vi "rsscope_core_global.vi"() -> ()   [LabVIEW 2014] (continued)
"Data Type"=0, "Command"="BUS{SerialBus}:DPHY:DPTW:SOUR", "Access"=2, "Range Table"="rsscope_rngWaveformParameter", "Read Callback"="", "Write Callback"="", "Supported Models"="", "Instrument Options"="K42", "Flags"=0, "Help"="Selects the source of the high speed data lane.\n\nAvailable Repeated Capabilities:\nSerialBus: SB1, SB2, SB3, SB4\r\n\nRemote-control command(s):\nBUS<m>:DPHY:DPTWo:SOURce"}, {"Level"=3, "Class Only"=FALSE, "Identifier"="RSSCOPE_ATTR_PROTOCOL_DPHY_DP_THREE_SOURCE", "Descriptive Name"="Protocol DPHY DP Three Source", "Data Type"=0, "Command"="BUS{SerialBus}:DPHY:DPTH:SOUR", "Access"=2, "Range Table"="rsscope_rngWaveformParameter", "Read Callback"="", "Write Callback"="", "Supported Models"="", "Instrument Options"="K42", "Flags"=0, "Help"="Selects the source of the high speed data lane.\n\nAvailable Repeated Capabilities:\nSerialBus: SB1, SB2, SB3, SB4\r\n\nRemote-control command(s):\nBUS<m>:DPHY:DPTHree:SOURce"}, {"Level"=3, "Class Only"=FALSE, "Identifier"="RSSCOPE_ATTR_PROTOCOL_DPHY_CP_PROBE", "Descriptive Name"="Protocol DPHY CP Probe", "Data Type"=0, "Command"="BUS{SerialBus}:DPHY:CP:PROB", "Access"=2, "Range Table"="rsscope_rngProbeDisplayDiff", "Read Callback"="", "Write Callback"="", "Supported Models"="", "Instrument Options"="", "Flags"=0, "Help"="Selects the type of probe used for the clock lane.\n\nAvailable Repeated Capabilities:\nSerialBus: SB1, SB2, SB3, SB4\r\n\nRemote-control command(s):\nBUS<m>:DPHY:CP:PROBe"}, {"Level"=3, "Class Only"=FALSE, "Identifier"="RSSCOPE_ATTR_PROTOCOL_DPHY_DN_ZERO_PROBE", "Descriptive Name"="Protocol DPHY DN Zero Probe", "Data Type"=0, "Command"="BUS{SerialBus}:DPHY:DNZ:PROB", "Access"=2, "Range Table"="rsscope_rngProbeDisplayDiff", "Read Callback"="", "Write Callback"="", "Supported Models"="", "Instrument Options"="K42", "Flags"=0, "Help"="Selects the type of probe used for the corresponding data lane.\n\nAvailable Repeated Capabilities:\nSerialBus: SB1, SB2, SB3, SB4\r\n\nRemote-control command(s):\nBUS<m>:DPHY:DNZero:PROBe"}, {"Level"=3, "Class Only"=FALSE, "Identifier"="RSSCOPE_ATTR_PROTOCOL_DPHY_DP_ZERO_PROBE", "Descriptive Name"="Protocol DPHY DP Zero Probe", "Data Type"=0, "Command"="BUS{SerialBus}:DPHY:DPZ:PROB", "Access"=2, "Range Table"="rsscope_rngProbeDisplayDiff", "Read Callback"="", "Write Callback"="", "Supported Models"="", "Instrument Options"="K42", "Flags"=0, "Help"="Selects the type of probe used for the corresponding data lane.\n\nAvailable Repeated Capabilities:\nSerialBus: SB1, SB2, SB3, SB4\r\n\nRemote-control command(s):\nBUS<m>:DPHY:DPZero:PROBe"}, {"Level"=3, "Class Only"=FALSE, "Identifier"="RSSCOPE_ATTR_PROTOCOL_DPHY_DP_ONE_PROBE", "Descriptive Name"="Protocol DPHY DP One Probe", "Data Type"=0, "Command"="BUS{SerialBus}:DPHY:DPON:PROB", "Access"=2, "Range Table"="rsscope_rngProbeDisplayDiff", "Read Callback"="", "Write Callback"="", "Supported Models"="", "Instrument Options"="K42", "Flags"=0, "Help"="Selects the type of probe used for the corresponding data lane.\n\nAvailable Repeated Capabilities:\nSerialBus: SB1, SB2, SB3, SB4\r\n\nRemote-control command(s):\nBUS<m>:DPHY:DPONe:PROBe"}, {"Level"=3, "Class Only"=FALSE, "Identifier"="RSSCOPE_ATTR_PROTOCOL_DPHY_DP_TWO_PROBE", "Descriptive Name"="Protocol DPHY DP Two Probe", "Data Type"=0, "Command"="BUS{SerialBus}:DPHY:DPTW:PROB", "Access"=2, "Range Table"="rsscope_rngProbeDisplayDiff", "Read Callback"="", "Write Callback"="", "Supported Models"="", "Instrument Options"="K42", "Flags"=0, "Help"="Selects the type of probe used for the corresponding data lane.\n\nAvailable Repeated Capabilities:\nSerialBus: SB1, SB2, SB3, SB4\r\n\nRemote-control command(s):\nBUS<m>:DPHY:DPTWo:PROBe"}, {"Level"=3, "Class Only"=FALSE, "Identifier"="RSSCOPE_ATTR_PROTOCOL_DPHY_DP_THREE_PROBE", "Descriptive Name"="Protocol DPHY DP Three Probe", "Data Type"=0, "Command"="BUS{SerialBus}:DPHY:DPTH:PROB", "Access"=2, "Range Table"="rsscope_rngProbeDisplayDiff", "Read Callback"="", "Write Callback"="", "Supported Models"="", "Instrument Options"="K42", "Flags"=0, "Help"="Selects the type of probe used for the corresponding data lane.\n\nAvailable Repeated Capabilities:\nSerialBus: SB1, SB2, SB3, SB4\r\n\nRemote-control command(s):\nBUS<m>:DPHY:DPTHree:PROBe"}, {"Level"=3, "Class Only"=FALSE, "Identifier"="RSSCOPE_ATTR_PROTOCOL_DPHY_DATA_RATE", "Descriptive Name"="Protocol DPHY Data Rate", "Data Type"=1, "Command"="BUS{SerialBus}:DPHY:DRAT", "Access"=2, "Range Table"="RsScope_rngDPHYDataRate", "Read Callback"="", "Write Callback"="", "Supported Models"="", "Instrument Options"="K42", "Flags"=0, "Help"="Sets a data rate.\n\nAvailable Repeated Capabilities:\nSerialBus: SB1, SB2, SB3, SB4\r\n\nRemote-control command(s):\nBUS<m>:DPHY:DRATe"}, {"Level"=3, "Class Only"=FALSE, "Identifier"="RSSCOPE_ATTR_PROTOCOL_DPHY_DISPALY_DATA_VECTOR", "Descriptive Name"="Protocol DPHY Dispaly Data Vector", "Data Type"=3, "Command"="BUS{SerialBus}:DPHY:DSPD", "Access"=2, "Range Table"="", "Read Callback"="", "Write Callback"="", "Supported Models"="", "Instrument Options"="K42", "Flags"=0, "Help"="Enables the display of the data vector, which means that the whole frame will be decoded.\nWhen the display vector is disabled only the packet header will be decoded and not the actual data payload of the frame. This will speed up the decoding.\n\nAvailable Repeated Capabilities:\nSerialBus: SB1, SB2, SB3, SB4\r\n\nRemote-control command(s):\nBUS<m>:DPHY:DSPData"}, {"Level"=3, "Class Only"=FALSE, "Identifier"="RSSCOPE_ATTR_PROTOCOL_DPHY_THRESHOLD_PRESET", "Descriptive Name"="Protocol DPHY Threshold Preset", "Data Type"=0, "Command"="BUS{SerialBus}:DPHY:THPR", "Access"=2, "Range Table"="RsScope_rngDPHYThresholdPreset", "Read Callback"="", "Write Callback"="", "Supported Models"="", "Instrument Options"="K42", "Flags"=0, "Help"="Prests the threshold and hysteresis values of the high speed data lanes. A preset sets the low power threshold to 1.20V and high speed threshold to 200 mV.\n\nAvailable Repeated Capabilities:\nSerialBus: SB1, SB2, SB3, SB4\r\n\nRemote-control command(s):\nBUS<m>:DPHY:THPReset"}, {"Level"=3, "Class Only"=FALSE, "Identifier"="RSSCOPE_ATTR_PROTOCOL_DPHY_THRESHOLD_COUPLING", "Descriptive Name"="Protocol DPHY Threshold Coupling", "Data Type"=3, "Command"="BUS{SerialBus}:DPHY:THC", "Access"=2, "Range Table"="", "Read Callback"="", "Write Callback"="", "Supported Models"="", "Instrument Options"="K42", "Flags"=0, "Help"="Enables coupling, i.e. the same threshold and hysteresis value is used for all lanes.\n\nAvailable Repeated Capabilities:\nSerialBus: SB1, SB2, SB3, SB4\r\n\nRemote-control command(s):\nBUS<m>:DPHY:THCoupling"}, {"Level"=3, "Class Only"=FALSE, "Identifier"="RSSCOPE_ATTR_PROTOCOL_DPHY_HIGH_SPEED_CP_THRESHOLD", "Descriptive Name"="Protocol DPHY High Speed CP Threshold", "Data Type"=1, "Command"="BUS{SerialBus}:DPHY:CP:HSP:THR", "Access"=2, "Range Table"="RsScope_rngDPHYHighSpeedThreshold", "Read Callback"="", "Write Callback"="", "Supported Models"="", "Instrument Options"="K42", "Flags"=0, "Help"="Sets the threshold value for the digitization of the respective high speed data line.\n\nAvailable Repeated Capabilities:\nSerialBus: SB1, SB2, SB3, SB4\r\n\nRemote-control command(s):\nBUS<m>:DPHY:CP:HSPeed:THReshold"}, {"Level"=3, "Class Only"=FALSE, "Identifier"="RSSCOPE_ATTR_PROTOCOL_DPHY_HIGH_SPEED_DP_ZERO_THRESHOLD", "Descriptive Name"="Protocol DPHY High Speed DP Zero Threshold", "Data Type"=1, "Command"="BUS{SerialBus}:DPHY:DPZ:HSP:THR", "Access"=2, "Range Table"="RsScope_rngDPHYHighSpeedThreshold", "Read Callback"="", "Write Callback"="", "Supported Models"="", "Instrument Options"="K42", "Flags"=0, "Help"="Sets the threshold value for the digitization of the respective high speed data line.\n\nAvailable Repeated Capabilities:\nSerialBus: SB1, SB2, SB3, SB4\r\n\nRemote-control command(s):\nBUS<m>:DPHY:DPZero:HSPeed:THReshold"}, {"Level"=3, "Class Only"=FALSE, "Identifier"="RSSCOPE_ATTR_PROTOCOL_DPHY_HIGH_SPEED_DP_ONE_THRESHOLD", "Descriptive Name"="Protocol DPHY High Speed DP One Threshold", "Data Type"=1, "Command"="BUS{SerialBus}:DPHY:DPON:HSP:THR", "Access"=2, "Range Table"="RsScope_rngDPHYHighSpeedThreshold", "Read Callback"="", "Write Callback"="", "Supported Models"="", "Instrument Options"="K42", "Flags"=0, "Help"="Sets the threshold value for the digitization of the respective high speed data line.\n\nAvailable Repeated Capabilities:\nSerialBus: SB1, SB2, SB3, SB4\r\n\nRemote-control command(s):\nBUS<m>:DPHY:DPONe:HSPeed:THReshold"}, {"Level"=3, "Class Only"=FALSE, "Identifier"="RSSCOPE_ATTR_PROTOCOL_DPHY_HIGH_SPEED_DP_TWO_THRESHOLD", "Descriptive Name"="Protocol DPHY High Speed DP Two Threshold", "Data Type"=1, "Command"="BUS{SerialBus}:DPHY:DPTW:HSP:THR", "Access"=2, "Range Table"="RsScope_rngDPHYHighSpeedThreshold", "Read Callback"="", "Write Callback"="", "Supported Models"="", "Instrument Options"="K42", "Flags"=0, "Help"="Sets the threshold value for the digitization of the respective high speed data line.\n\nAvailable Repeated Capabilities:\nSerialBus: SB1, SB2, SB3, SB4\r\n\nRemote-control command(s):\nBUS<m>:DPHY:DPTWo:HSPeed:THReshold"}, {"Level"=3, "Class Only"=FALSE, "Identifier"="RSSCOPE_ATTR_PROTOCOL_DPHY_HIGH_SPEED_DP_THREE_THRESHOLD", "Descriptive Name"="Protocol DPHY High Speed DP Three Threshold", "Data Type"=1, "Command"="BUS{SerialBus}:DPHY:DPTH:HSP:THR", "Access"=2, "Range Table"="RsScope_rngDPHYHighSpeedThreshold", "Read Callback"="", "Write Callback"="", "Supported Models"="", "Instrument Options"="K42", "Flags"=0, "Help"="Sets the threshold value for the digitization of the respective high speed data line.\n\nAvailable Repeated Capabilities:\nSerialBus: SB1, SB2, SB3, SB4\r\n\nRemote-control command(s):\nBUS<m>:DPHY:DPTHree:HSPeed:THReshold"}, {"Level"=3, "Class Only"=FALSE, "Identifier"="RSSCOPE_ATTR_PROTOCOL_DPHY_HIGH_SPEED_CP_HYSTERESIS", "Descriptive Name"="Protocol DPHY High Speed CP Hysteresis", "Data Type"=1, "Command"="BUS{SerialBus}:DPHY:CP:HSP:HYST", "Access"=2, "Range Table"="RsScope_rngDPHYHighSpeedHysteresis", "Read Callback"="", "Write Callback"="", "Supported Models"="", "Instrument Options"="K42", "Flags"=0, "Help"="Sets a value for the hysteresis of the respective lane.\n\nAvailable Repeated Capabilities:\nSerialBus: SB1, SB2, SB3, SB4\r\n\nRemote-control command(s):\nBUS<m>:DPHY:CP:HSPeed:HYSTeresis"}, {"Level"=3, "Class Only"=FALSE, "Identifier"="RSSCOPE_ATTR_PROTOCOL_DPHY_HIGH_SPEED_DP_ZERO_HYSTERESIS", "Descriptive Name"="Protocol DPHY High Speed DP Zero Hysteresis", "Data Type"=1, "Command"="BUS{SerialBus}:DPHY:DPZ:HSP:HYST", "Access"=2, "Range Table"="RsScope_rngDPHYHighSpeedHysteresis", "Read Callback"="", "Write Callback"="", "Supported Models"="", "Instrument Options"="K42", "Flags"=0, "Help"="Sets a value for the hysteresis of the respective lane.\n\nAvailable Repeated Capabilities:\nSerialBus: SB1, SB2, SB3, SB4\r\n\nRemote-control command(s):\nBUS<m>:DPHY:DPZero:HSPeed:HYSTeresis"}, {"Level"=3, "Class Only"=FALSE, "Identifier"="RSSCOPE_ATTR_PROTOCOL_DPHY_HIGH_SPEED_DP_ONE_HYSTERESIS", "Descriptive Name"="Protocol DPHY High Speed DP One Hysteresis", "Data Type"=1, "Command"="BUS{SerialBus}:DPHY:DPON:HSP:HYST", "Access"=2, "Range Table"="RsScope_rngDPHYHighSpeedHysteresis", "Read Callback"="", "Write Callback"="", "Supported Models"="", "Instrument Options"="K42", "Flags"=0, "Help"="Sets a value for the hysteresis of the respective lane.\n\nAvailable Repeated Capabilities:\nSerialBus: SB1, SB2, SB3, SB4\r\n\nRemote-control command(s):\nBUS<m>:DPHY:DPONe:HSPeed:HYSTeresis"}, {"Level"=3, "Class Only"=FALSE, "Identifier"="RSSCOPE_ATTR_PROTOCOL_DPHY_HIGH_SPEED_DP_TWO_HYSTERESIS", "Descriptive Name"="Protocol DPHY High Speed DP Two Hysteresis", "Data Type"=1, "Command"="BUS{SerialBus}:DPHY:DPTW:HSP:HYST", "Access"=2, "Range Table"="RsScope_rngDPHYHighSpeedHysteresis", "Read Callback"="", "Write Callback"="", "Supported Models"="", "Instrument Options"="K42", "Flags"=0, "Help"="Sets a value for the hysteresis of the respective lane.\n\nAvailable Repeated Capabilities:\nSerialBus: SB1, SB2, SB3, SB4\r\n\nRemote-control command(s):\nBUS<m>:DPHY:DPTWo:HSPeed:HYSTeresis"}, {"Level"=3, "Class Only"=FALSE, "Identifier"="RSSCOPE_ATTR_PROTOCOL_DPHY_HIGH_SPEED_DP_THREE_HYSTERESIS", "Descriptive Name"="Protocol DPHY High Speed DP Three Hysteresis", "Data Type"=1, "Command"="BUS{SerialBus}:DPHY:DPTH:HSP:HYST", "Access"=2, "Range Table"="RsScope_rngDPHYHighSpeedHysteresis", "Read Callback"="", "Write Callback"="", "Supported Models"="", "Instrument Options"="K42", "Flags"=0, "Help"="Sets a value for the hysteresis of the respective lane.\n\nAvailable Repeated Capabilities:\nSerialBus: SB1, SB2, SB3, SB4\r\n\nRemote-control command(s):\nBUS<m>:DPHY:DPTHree:HSPeed:HYSTeresis"}, {"Level"=3, "Class Only"=FALSE, "Identifier"="RSSCOPE_ATTR_PROTOCOL_DPHY_LOW_POWER_DN_ZERO_THRESHOLD_UPPER", "Descriptive Name"="Protocol DPHY Low Power DN Zero Threshold Upper", "Data Type"=1, "Command"="BUS{SerialBus}:DPHY:DNZ:LPOW:THUP", "Access"=2, "Range Table"="RsScope_rnglDPHYLowPowerThreshold", "Read Callback"="", "Write Callback"="", "Supported Models"="", "Instrument Options"="K42", "Flags"=0, "Help"="Sets the upper threshold value for the respective lane used for the low power mode.\n\nAvailable Repeated Capabilities:\nSerialBus: SB1, SB2, SB3, SB4\r\n\nRemote-control command(s):\nBUS<m>:DPHY:DNZero:LPOWer:THUPper"}, {"Level"=3, "Class Only"=FALSE, "Identifier"="RSSCOPE_ATTR_PROTOCOL_DPHY_LOW_POWER_DP_ZERO_THRESHOLD_UPPER", "Descriptive Name"="Protocol DPHY Low Power DP Zero Threshold Upper", "Data Type"=1, "Command"="BUS{SerialBus}:DPHY:DPZ:LPOW:THUP", "Access"=2, "Range Table"="RsScope_rnglDPHYLowPowerThreshold", "Read Callback"="", "Write Callback"="", "Supported Models"="", "Instrument Options"="K42", "Flags"=0, "Help"="Sets the upper threshold value for the respective lane used for the low power mode.\n\nAvailable Repeated Capabilities:\nSerialBus: SB1, SB2, SB3, SB4\r\n\nRemote-control command(s):\nBUS<m>:DPHY:DPZero:LPOWer:THUPper"}, {"Level"=3, "Class Only"=FALSE, "Identifier"="RSSCOPE_ATTR_PROTOCOL_DPHY_LOW_POWER_DN_ZERO_THRESHOLD_LOWER", "Descriptive Name"="Protocol DPHY Low Power DN Zero Threshold Lower", "Data Type"=1, "Command"="BUS{SerialBus}:DPHY:DNZ:LPOW:THL", "Access"=2, "Range Table"="RsScope_rnglDPHYLowPowerThreshold", "Read Callback"="", "Write Callback"="", "Supported Models"="", "Instrument Options"="K42", "Flags"=0, "Help"="Sets the lower threshold value for the respective lane used for the low power mode.\n\nAvailable Repeated Capabilities:\nSerialBus: SB1, SB2, SB3, SB4\r\n\nRemote-control command(s):\nBUS<m>:DPHY:DNZero:LPOWer:THLower"}, {"Level"=3, "Class Only"=FALSE, "Identifier"="RSSCOPE_ATTR_PROTOCOL_DPHY_LOW_POWER_DP_ZERO_THRESHOLD_LOWER", "Descriptive Name"="Protocol DPHY Low Power DP Zero Threshold Lower", "Data Type"=1, "Command"="BUS{SerialBus}:DPHY:DPZ:LPOW:THL", "Access"=2, "Range Table"="RsScope_rnglDPHYLowPowerThreshold", "Read Callback"="", "Write Callback"="", "Supported Models"="", "Instrument Options"="K42", "Flags"=0, "Help"="Sets the lower threshold value for the respective lane used for the low power mode.\n\nAvailable Repeated Capabilities:\nSerialBus: SB1, SB2, SB3, SB4\r\n\nRemote-control command(s):\nBUS<m>:DPHY:DPZero:LPOWer:THLower"}, {"Level"=3, "Class Only"=FALSE, "Identifier"="RSSCOPE_ATTR_PROTOCOL_DPHY_SHOW_MULTIPLE_LANES", "Descriptive Name"="Protocol DPHY Show Multiple Lanes", "Data Type"=3, "Command"="BUS{SerialBus}:DPHY:SML", "Access"=2, "Range Table"="", "Read Callback"="", "Write Callback"="", "Supported Models"="", "Instrument Options"="K42", "Flags"=0, "Help"="Enables the display of the results in multiple lanes.\n\nAvailable Repeated Capabilities:\nSerialBus: SB1, SB2, SB3, SB4\r\n\nRemote-control command(s):\nBUS<m>:DPHY:SMLanes"}, {"Level"=3, "Class Only"=TRUE, "Identifier"="", "Descriptive Name"="Decoding Results", "Data Type"=0, "Command"="", "Access"=0, "Range Table"="", "Read Callback"="", "Write Callback"="", "Supported Models"="", "Instrument Options"="", "Flags"=0, "Help"="Returns the D-PHY decoding results."}, {"Level"=4, "Class Only"=FALSE, "Identifier"="RSSCOPE_ATTR_PROTOCOL_DPHY_FRAME_COUNT", "Descriptive Name"="Protocol DPHY Frame Count", "Data Type"=0, "Command"="BUS{SerialBus}:DPHY:RES:FCO?", "Access"=0, "Range Table"="", "Read Callback"="", "Write Callback"="", "Supported Models"="", "Instrument Options"="K42", "Flags"=0, "Help"="Returns the number of decoded frames for the selected serial bus.\n\nAvailable Repeated Capabilities:\nSerialBus: SB1, SB2, SB3, SB4\r\n\nRemote-control command(s):\nBUS<m>:DPHY:RESult:FCOunt?"}, {"Level"=2, "Class Only"=TRUE, "Identifier"="", "Descriptive Name"="M-PHY", "Data Type"=0, "Command"="", "Access"=0, "Range Table"="", "Read Callback"="", "Write Callback"="", "Supported Models"="", "Instrument Options"="", "Flags"=0, "Help"="Contains attributes for M-PHY."}, {"Level"=3, "Class Only"=FALSE, "Identifier"="RSSCOPE_ATTR_PROTOCOL_MPHY", "Descriptive Name"="Protocol MPHY", "Data Type"=0, "Command"="BUS{SerialBus}:MPHY:VAR", "Access"=2, "Range Table"="RsScope_rngProtocolMPHY", "Read Callback"="", "Write Callback"="", "Supported Models"="", "Instrument Options"="", "Flags"=0, "Help"="Selects the protocol running on the interface.\n\nAvailable Repeated Capabilities:\nSerialBus: SB1, SB2, SB3, SB4\r\n\nRemote-control command(s):\nBUS<m>:MPHY:VARiant"}, {"Level"=3, "Class Only"=FALSE, "Identifier"="RSSCOPE_ATTR_PROTOCOL_MPHY_DATA_LANES", "Descriptive Name"="Protocol MPHY Data Lanes", "Data Type"=0, "Command"="BUS{SerialBus}:MPHY:DLAN", "Access"=2, "Range Table"="RsScope_rngDPHYDataLanes", "Read Callback"="", "Write Callback"="", "Supported Models"="", "Instrument Options"="", "Flags"=0, "Help"="Sets the number of data lanes.\n\nAvailable Repeated Capabilities:\nSerialBus: SB1, SB2, SB3, SB4\r\n\nRemote-control command(s):\nBUS<m>:MPHY:DLANes"}, {"Level"=3, "Class Only"=FALSE, "Identifier"="RSSCOPE_ATTR_PROTOCOL_MPHY_DATA_SOURCE_ZERO", "Descriptive Name"="Protocol MPHY Data Source Zero", "Data Type"=0, "Command"="BUS{SerialBus}:MPHY:DZER:SOUR", "Access"=2, "Range Table"="RsScope_rngMPHYDataSource", "Read Callback"="", "Write Callback"="", "Supported Models"="", "Instrument Options"="", "Flags"=0, "Help"="Selects the source of the corresponding data lane.\n\nAvailable Repeated Capabilities:\nSerialBus: SB1, SB2, SB3, SB4\r\n\nRemote-control command(s):\nBUS<m>:MPHY:DZERo:SOURce"}, {"Level"=3, "Class Only"=FALSE, "Identifier"="RSSCOPE_ATTR_PROTOCOL_MPHY_DATA_SOURCE_ONE", "Descriptive Name"="Protocol MPHY Data Source One", "Data Type"=0, "Command"="BUS{SerialBus}:MPHY:DONE:SOUR", "Access"=2, "Range Table"="RsScope_rngMPHYDataSource", "Read Callback"="", "Write Callback"="", "Supported Models"="", "Instrument Options"="", "Flags"=0, "Help"="Selects the source of the corresponding data lane.\n\nAvailable Repeated Capabilities:\nSerialBus: SB1, SB2, SB3, SB4\r\n\nRemote-control command(s):\nBUS<m>:MPHY:DONE:SOURce"}, {"Level"=3, "Class Only"=FALSE, "Identifier"="RSSCOPE_ATTR_PROTOCOL_MPHY_DATA_SOURCE_TWO", "Descriptive Name"="Protocol MPHY Data Source Two", "Data Type"=0, "Command"="BUS{SerialBus}:MPHY:DTWO:SOUR", "Access"=2, "Range Table"="RsScope_rngMPHYDataSource", "Read Callback"="", "Write Callback"="", "Supported Models"="", "Instrument Options"="K44", "Flags"=0, "Help"="Selects the source of the corresponding data lane.\n\nAvailable Repeated Capabilities:\nSerialBus: SB1, SB2, SB3, SB4\r\n\nRemote-control command(s):\nBUS<m>:MPHY:DTWO:SOURce"}, {"Level"=3, "Class Only"=FALSE, "Identifier"="RSSCOPE_ATTR_PROTOCOL_MPHY_DATA_SOURCE_THREE", "Descriptive Name"="Protocol MPHY Data Source Three", "Data Type"=0, "Command"="BUS{SerialBus}:MPHY:DTHR:SOUR", "Access"=2, "Range Table"="RsScope_rngMPHYDataSource", "Read Callback"="", "Write Callback"="", "Supported Models"="", "Instrument Options"="K44", "Flags"=0, "Help"="Selects the source of the corresponding data lane.\n\nAvailable Repeated Capabilities:\nSerialBus: SB1, SB2, SB3, SB4\r\n\nRemote-control command(s):\nBUS<m>:MPHY:DTHRee:SOURce"}, {"Level"=3, "Class Only"=FALSE, "Identifier"="RSSCOPE_ATTR_PROTOCOL_MPHY_THRESHOLD_ZERO", "Descriptive Name"="Protocol MPHY Threshold Zero", "Data Type"=1, "Command"="BUS{SerialBus}:MPHY:DZER:THR", "Access"=2, "Range Table"="RsScope_rngMPHYThreshold", "Read Callback"="", "Write Callback"="", "Supported Models"="", "Instrument Options"="K44", "Flags"=0, "Help"="Sets the threshold value for the respective lane.\n\nAvailable Repeated Capabilities:\nSerialBus: SB1, SB2, SB3, SB4\r\n\nRemote-control command(s):\nBUS<m>:MPHY:DZERo:THReshold"}, {"Level"=3, "Class Only"=FALSE, "Identifier"="RSSCOPE_ATTR_PROTOCOL_MPHY_THRESHOLD_ONE", "Descriptive Name"="Protocol MPHY Threshold One", "Data Type"=1, "Command"="BUS{SerialBus}:MPHY:DONE:THR", "Access"=2, "Range Table"="RsScope_rngMPHYThreshold", "Read Callback"="", "Write Callback"="", "Supported Models"="", "Instrument Options"="K44", "Flags"=0, "Help"="Sets the threshold value for the respective lane.\n\nAvailable Repeated Capabilities:\nSerialBus: SB1, SB2, SB3, SB4\r\n\nRemote-control command(s):\nBUS<m>:MPHY:DONE:THReshold"}, {"Level"=3, "Class Only"=FALSE, "Identifier"="RSSCOPE_ATTR_PROTOCOL_MPHY_THRESHOLD_TWO", "Descriptive Name"="Protocol MPHY Threshold Two", "Data Type"=1, "Command"="BUS{SerialBus}:MPHY:DTWO:THR", "Access"=2, "Range Table"="RsScope_rngMPHYThreshold", "Read Callback"="", "Write Callback"="", "Supported Models"="", "Instrument Options"="K44", "Flags"=0, "Help"="Sets the threshold value for the respective lane.\n\nAvailable Repeated Capabilities:\nSerialBus: SB1, SB2, SB3, SB4\r\n\nRemote-control command(s):\nBUS<m>:MPHY:DTWO:THReshold"}, {"Level"=3, "Class Only"=FALSE, "Identifier"="RSSCOPE_ATTR_PROTOCOL_MPHY_THRESHOLD_THREE", "Descriptive Name"="Protocol MPHY Threshold Three", "Data Type"=1, "Command"="BUS{SerialBus}:MPHY:DTHR:THR", "Access"=2, "Range Table"="RsScope_rngMPHYThreshold", "Read Callback"="", "Write Callback"="", "Supported Models"="", "Instrument Options"="K44", "Flags"=0, "Help"="Sets the threshold value for the respective lane.\n\nAvailable Repeated Capabilities:\nSerialBus: SB1, SB2, SB3, SB4\r\n\nRemote-control command(s):\nBUS<m>:MPHY:DTHRee:THReshold"}, {"Level"=3, "Class Only"=FALSE, "Identifier"="RSSCOPE_ATTR_PROTOCOL_MPHY_THRESHOLD_COUPLING_ENABLED", "Descriptive Name"="Protocol MPHY Threshold Coupling Enabled", "Data Type"=3, "Command"="BUS{SerialBus}:MPHY:THC", "Access"=2, "Range Table"="", "Read Callback"="", "Write Callback"="", "Supported Models"="", "Instrument Options"="K44", "Flags"=0, "Help"="Enables the same threshold value to be used for all lanes.\nWhen the threshold coupling is disabled, changes to the threshold value only affect the respective lane.\n\nAvailable Repeated Capabilities:\nSerialBus: SB1, SB2, SB3, SB4\r\n\nRemote-control command(s):\nBUS<m>:MPHY:THCoupling"}, {"Level"=3, "Class Only"=FALSE, "Identifier"="RSSCOPE_ATTR_PROTOCOL_MPHY_THRESHOLD_PRESET", "Descriptive Name"="Protocol MPHY Threshold Preset", "Data Type"=0, "Command"="BUS{SerialBus}:MPHY:THPR", "Access"=2, "Range Table"="RsScope_rngMPHYThresholdPreset", "Read Callback"="", "Write Callback"="", "Supported Models"="", "Instrument Options"="K44", "Flags"=0, "Help"="Selects the predefined value to preset the threshold value of the data lanes.\n\nAvailable Repeated Capabilities:\nSerialBus: SB1, SB2, SB3, SB4\r\n\nRemote-control command(s):\nBUS<m>:MPHY:THPReset"}, {"Level"=3, "Class Only"=FALSE, "Identifier"="RSSCOPE_ATTR_PROTOCOL_MPHY_SCRAMBLED_MODE", "Descriptive Name"="Protocol MPHY Scrambled Mode", "Data Type"=0, "Command"="BUS{SerialBus}:MPHY:SCRM", "Access"=2, "Range Table"="RsScope_rngMPHYScrambleMode", "Read Callback"="", "Write Callback"="", "Supported Models"="", "Instrument Options"="K44", "Flags"=0, "Help"="Sets if the SSIC data is scrambled or unscrambled.\n\nAvailable Repeated Capabilities:\nSerialBus: SB1, SB2, SB3, SB4\r\n\nRemote-control command(s):\nBUS<m>:MPHY:SCRMode"}, {"Level"=3, "Class Only"=FALSE, "Identifier"="RSSCOPE_ATTR_PROTOCOL_MPHY_SHOW_MULTIPLE_LANES", "Descriptive Name"="Protocol MPHY Show Multiple Lanes", "Data Type"=3, "Command"="BUS{SerialBus}:MPHY:SML", "Access"=2, "Range Table"="", "Read Callback"="", "Write Callback"="", "Supported Models"="", "Instrument Options"="K44", "Flags"=0, "Help"="Enables the display of the results in multiple lanes.\n\nAvailable Repeated Capabilities:\nSerialBus: SB1, SB2, SB3, SB4\r\n\nRemote-control command(s):\nBUS<m>:MPHY:SMLanes"}, {"Level"=3, "Class Only"=TRUE, "Identifier"="", "Descriptive Name"="Decoding Results", "Data Type"=0, "Command"="", "Access"=0, "Range Table"="", "Read Callback"="", "Write Callback"="", "Supported Models"="", "Instrument Options"="", "Flags"=0, "Help"="Returns the M-PHY decoding results."}, {"Level"=4, "Class Only"=FALSE, "Identifier"="RSSCOPE_ATTR_PROTOCOL_MPHY_FRAME_COUNT", "Descriptive Name"="Protocol MPHY Frame Count", "Data Type"=0, "Command"="BUS{SerialBus}:MPHY:RES:FCO?", "Access"=0, "Range Table"="", "Read Callback"="", "Write Callback"="", "Supported Models"="", "Instrument Options"="K44", "Flags"=0, "Help"="Returns the number of decoded frames.\n\nAvailable Repeated Capabilities:\nSerialBus: SB1, SB2, SB3, SB4\r\n\nRemote-control command(s):\nBUS<m>:MPHY:RESult:FCOunt?"}, {"Level"=2, "Class Only"=TRUE, "Identifier"="", "Descriptive Name"="Space Wire", "Data Type"=0, "Command"="", "Access"=0, "Range Table"="", "Read Callback"="", "Write Callback"="", "Supported Models"="", "Instrument Options"="", "Flags"=0, "Help"="The SpaceWire (K65) is a communication network standard used for spacecrafts. It is based on the IEEE 1355 standard of comunications and coordinated by the European Space Agency (ESA)."}, {"Level"=3, "Class Only"=FALSE, "Identifier"="RSSCOPE_ATTR_PROTOCOL_SPACE_WIRE_STROBE_SOURCE", "Descriptive Name"="Protocol Space Wire Strobe Source", "Data Type"=0, "Command"="BUS{SerialBus}:SWIR:STRB:SOUR", "Access"=2, "Range Table"="rsscope_rngWaveformParameter", "Read Callback"="", "Write Callback"="", "Supported Models"="", "Instrument Options"="K65", "Flags"=0, "Help"="Selects the source of the strobe signal.\n\nAvailable Repeated Capabilities:\nSerialBus: SB1, SB2, SB3, SB4\r\n\nRemote-control command(s):\nBUS<m>:SWIRe:STRBe:SOURce"}, {"Level"=3, "Class Only"=FALSE, "Identifier"="RSSCOPE_ATTR_PROTOCOL_SPACE_WIRE_DATA_SOURCE", "Descriptive Name"="Protocol Space Wire Data Source", "Data Type"=0, "Command"="BUS{SerialBus}:SWIR:DATA:SOUR", "Access"=2, "Range Table"="rsscope_rngWaveformParameter", "Read Callback"="", "Write Callback"="", "Supported Models"="", "Instrument Options"="K65", "Flags"=0, "Help"="Selects the source of the data signal.\n\nAvailable Repeated Capabilities:\nSerialBus: SB1, SB2, SB3, SB4\r\n\nRemote-control command(s):\nBUS<m>:SWIRe:DATA:SOURce"}, {"Level"=3, "Class Only"=FALSE, "Identifier"="RSSCOPE_ATTR_PROTOCOL_SPACE_WIRE_THRESHOLD_PRESET", "Descriptive Name"="Protocol Space Wire Threshold Preset", "Data Type"=0, "Command"="BUS{SerialBus}:SWIR:PRES", "Access"=2, "Range Table"="RsScope_rngSpaceWireThresholdPreset", "Read Callback"="", "Write Callback"="", "Supported Models"="", "Instrument Options"="K65", "Flags"=0, "Help"="Presets the threshold and hysteresis value of the strobe and data signal.\n\nAvailable Repeated Capabilities:\nSerialBus: SB1, SB2, SB3, SB4\r\n\nRemote-control command(s):\nBUS<m>:SWIRe:PRESet"}, {"Level"=3, "Class Only"=FALSE, "Identifier"="RSSCOPE_ATTR_PROTOCOL_SPACE_WIRE_THRESHOLD_COUPLING", "Descriptive Name"="Protocol Space Wire Threshold Coupling", "Data Type"=3, "Command"="BUS{SerialBus}:SWIR:COUP", "Access"=2, "Range Table"="", "Read Callback"="", "Write Callback"="", "Supported Models"="", "Instrument Options"="K65", "Flags"=0, "Help"="Enables coupling, i.e. the same threshold and hysteresis value is used for the strob and the data signal.\n\nAvailable Repeated Capabilities:\nSerialBus: SB1, SB2, SB3, SB4\r\n\nRemote-control command(s):\nBUS<m>:SWIRe:COUPling"}, {"Level"=3, "Class Only"=FALSE, "Identifier"="RSSCOPE_ATTR_PROTOCOL_SPACE_WIRE_STROBE_THRESHOLD", "Descriptive Name"="Protocol Space Wire Strobe Threshold", "Data Type"=1, "Command"="BUS{SerialBus}:SWIR:STRB:THR", "Access"=2, "Range Table"="RsScope_rngSpaceWireThreshold", "Read Callback"="", "Write Callback"="", "Supported Models"="", "Instrument Options"="K65", "Flags"=0, "Help"="Sets the threshold value for the digitization of the strobe signal.\n\nAvailable Repeated Capabilities:\nSerialBus: SB1, SB2, SB3, SB4\r\n\nRemote-control command(s):\nBUS<m>:SWIRe:STRBe:THReshold"}, {"Level"=3, "Class Only"=FALSE, "Identifier"="RSSCOPE_ATTR_PROTOCOL_SPACE_WIRE_DATA_THRESHOLD", "Descriptive Name"="Protocol Space Wire Data Threshold", "Data Type"=1, "Command"="BUS{SerialBus}:SWIR:DATA:THR", "Access"=2, "Range Table"="RsScope_rngSpaceWireThreshold", "Read Callback"="", "Write Callback"="", "Supported Models"="", "Instrument Options"="K65", "Flags"=0, "Help"="Sets the threshold value for the digitization of the data signal.\n\nAvailable Repeated Capabilities:\nSerialBus: SB1, SB2, SB3, SB4\r\n\nRemote-control command(s):\nBUS<m>:SWIRe:DATA:THReshold"}, {"Level"=3, "Class Only"=FALSE, "Identifier"="RSSCOPE_ATTR_PROTOCOL_SPACE_WIRE_STROBE_HYSTERESIS", "Descriptive Name"="Protocol Space Wire Strobe Hysteresis", "Data Type"=1, "Command"="BUS{SerialBus}:SWIR:STRB:HYST", "Access"=2, "Range Table"="RsScope_rngSpaceWireHysteresis", "Read Callback"="", "Write Callback"="", "Supported Models"="", "Instrument Options"="K65", "Flags"=0, "Help"="Sets a value for the hysteresis of the strobe signal.\n\nAvailable Repeated Capabilities:\nSerialBus: SB1, SB2, SB3, SB4\r\n\nRemote-control command(s):\nBUS<m>:SWIRe:STRBe:HYSTeresis"}, {"Level"=3, "Class Only"=FALSE, "Identifier"="RSSCOPE_ATTR_PROTOCOL_SPACE_WIRE_DATA_HYSTERESIS", "Descriptive Name"="Protocol Space Wire Data Hysteresis", "Data Type"=1, "Command"="BUS{SerialBus}:SWIR:DATA:HYST", "Access"=2, "Range Table"="RsScope_rngSpaceWireHysteresis", "Read Callback"="", "Write Callback"="", "Supported Models"="", "Instrument Options"="K65", "Flags"=0, "Help"="Sets a value for the hysteresis of the data signal.\n\nAvailable Repeated Capabilities:\nSerialBus: SB1, SB2, SB3, SB4\r\n\nRemote-control command(s):\nBUS<m>:SWIRe:DATA:HYSTeresis"}, {"Level"=3, "Class Only"=FALSE, "Identifier"="RSSCOPE_ATTR_PROTOCOL_SPACE_WIRE_SYNC_SETTINGS", "Descriptive Name"="Protocol Space Wire Sync Settings", "Data Type"=0, "Command"="BUS{SerialBus}:SWIR:SYSL", "Access"=2, "Range Table"="rsscope_rngAutoManual", "Read Callback"="", "Write Callback"="", "Supported Models"="", "Instrument Options"="K65", "Flags"=0, "Help"="Selects the mode for the synchronisation settings, i.e i.e. packet align.\n\nAvailable Repeated Capabilities:\nSerialBus: SB1, SB2, SB3, SB4\r\n\nRemote-control command(s):\nBUS<m>:SWIRe:SYSLect"}, {"Level"=3, "Class Only"=FALSE, "Identifier"="RSSCOPE_ATTR_PROTOCOL_SPACE_WIRE_SYNC_BIT_POSITION", "Descriptive Name"="Protocol Space Wire Sync Bit Position", "Data Type"=0, "Command"="BUS{SerialBus}:SWIR:BPOS", "Access"=2, "Range Table"="RsScope_rngSpaceWireSyncBitPosition", "Read Callback"="", "Write Callback"="", "Supported Models"="", "Instrument Options"="K65", "Flags"=0, "Help"="Sets the bit position, the align position for the manual synchronisation mode. This can be useful when parity errors exist in the signal, and parity check is the main indicator for the decoder to do packet alignment.\n\nAvailable Repeated Capabilities:\nSerialBus: SB1, SB2, SB3, SB4\r\n\nRemote-control command(s):\nBUS<m>:SWIRe:BPOSition"}, {"Level"=3, "Class Only"=FALSE, "Identifier"="RSSCOPE_ATTR_PROTOCOL_SPACE_WIRE_MIN_GAP", "Descriptive Name"="Protocol Space Wire Min Gap", "Data Type"=1, "Command"="BUS{SerialBus}:SWIR:MGAP", "Access"=2, "Range Table"="RsScope_rngSpaceWireMinGap", "Read Callback"="", "Write Callback"="", "Supported Models"="", "Instrument Options"="K65", "Flags"=0, "Help"="Sets the minimum duration of a gap. Any inactivity greater than this time will be interpreted as a gap and lead to a resynchronization to the signal.\n\nAvailable Repeated Capabilities:\nSerialBus: SB1, SB2, SB3, SB4\r\n\nRemote-control command(s):\nBUS<m>:SWIRe:MGAP"}, {"Level"=3, "Class Only"=TRUE, "Identifier"="", "Descriptive Name"="Decoding Results", "Data Type"=0, "Command"="", "Access"=0, "Range Table"="", "Read Callback"="", "Write Callback"="", "Supported Models"="", "Instrument Options"="", "Flags"=0, "Help"="Returns the Space Wire decoding results."}, {"Level"=4, "Class Only"=FALSE, "Identifier"="RSSCOPE_ATTR_PROTOCOL_SPACE_WIRE_FRAME_COUNT", "Descriptive Name"="Protocol Space Wire Frame Count", "Data Type"=0, "Command"="BUS{SerialBus}:SWIR:RES:FCO?", "Access"=0, "Range Table"="", "Read Callback"="", "Write Callback"="", "Supported Models"="", "Instrument Options"="K65", "Flags"=0, "Help"="Returns the number of decoded frames for the selected serial bus.\n\nAvailable Repeated Capabilities:\nSerialBus: SB1, SB2, SB3, SB4\r\n\nRemote-control command(s):\nBUS<m>:SWIRe:RESults:FCOunt?"}, {"Level"=2, "Class Only"=TRUE, "Identifier"="", "Descriptive Name"="CXPI", "Data Type"=0, "Command"="", "Access"=0, "Range Table"="", "Read Callback"="", "Write Callback"="", "Supported Models"="", "Instrument Options"="", "Flags"=0, "Help"="Main characteristics of CXPI are:\nCarrier Sense Multiple Access (CSMA) and Collision Resolution (CR).\nThe master sends pulse width modulated clock (PWMC).\nSupport of the sleep/wake function to reduce power consumption.\nSupport of two methods for frame transfer management, the event trigger method and the polling method.\nThe event trigger method can be used when the focus is placed on the responsiveness of the slave node communication. The polling method puts the focus on the communication periodicity.\nMaximum baud rate of 20kbit/s.\nUp to 16 nodes connected to a communication bus"}, {"Level"=3, "Class Only"=FALSE, "Identifier"="RSSCOPE_ATTR_PROTOCOL_CXPI_SOURCE", "Descriptive Name"="Protocol CXPI Source", "Data Type"=0, "Command"="BUS{SerialBus}:CXPI:SDAT", "Access"=2, "Range Table"="rsscope_rngProtocolWaveformSource", "Read Callback"="", "Write Callback"="", "Supported Models"="", "Instrument Options"="K76", "Flags"=0, "Help"="Selects the source of the strobe signal.\n\nAvailable Repeated Capabilities:\nSerialBus: SB1, SB2, SB3, SB4\r\n\nRemote-control command(s):\nBUS<m>:CXPI:SDATa"}, {"Level"=3, "Class Only"=FALSE, "Identifier"="RSSCOPE_ATTR_PROTOCOL_CXPI_POLARITY", "Descriptive Name"="Protocol CXPI Polarity", "Data Type"=0, "Command"="BUS{SerialBus}:CXPI:POL", "Access"=2, "Range Table"="rsscope_rngCXPIPolarity", "Read Callback"="", "Write Callback"="", "Supported Models"="", "Instrument Options"="K76", "Flags"=0, "Help"="Sets the polarity of the transmitted waveform to normal (high = 1) or inverted (low = 1).\n\nAvailable Repeated Capabilities:\nSerialBus: SB1, SB2, SB3, SB4\r\n\nRemote-control command(s):\nBUS<m>:CXPI:POLarity"}, {"Level"=3, "Class Only"=FALSE, "Identifier"="RSSCOPE_ATTR_PROTOCOL_CXPI_THRESHOLD", "Descriptive Name"="Protocol CXPI Threshold", "Data Type"=1, "Command"="BUS{SerialBus}:CXPI:THR", "Access"=2, "Range Table"="RsScope_rngCXPIThreshold", "Read Callback"="", "Write Callback"="", "Supported Models"="", "Instrument Options"="K76", "Flags"=0, "Help"="Sets the threshold value for the signal.\n\nAvailable Repeated Capabilities:\nSerialBus: SB1, SB2, SB3, SB4\r\n\nRemote-control command(s):\nBUS<m>:CXPI:THReshold"}, {"Level"=3, "Class Only"=FALSE, "Identifier"="RSSCOPE_ATTR_PROTOCOL_CXPI_HYSTERESIS", "Descriptive Name"="Protocol CXPI Hysteresis", "Data Type"=1, "Command"="BUS{SerialBus}:CXPI:HYST", "Access"=2, "Range Table"="RsScope_rngCXPIHysteresis", "Read Callback"="", "Write Callback"="", "Supported Models"="", "Instrument Options"="K76", "Flags"=0, "Help"="Sets a value for the hysteresis.\n\nAvailable Repeated Capabilities:\nSerialBus: SB1, SB2, SB3, SB4\r\n\nRemote-control command(s):\nBUS<m>:CXPI:HYSTeresis"}, {"Level"=3, "Class Only"=FALSE, "Identifier"="RSSCOPE_ATTR_PROTOCOL_CXPI_DISPLAY_ORDER", "Descriptive Name"="Protocol CXPI Display Order", "Data Type"=0, "Command"="BUS{SerialBus}:CXPI:DORD", "Access"=2, "Range Table"="RsScope_rngCXPIDisplayOrder", "Read Callback"="", "Write Callback"="", "Supported Models"="", "Instrument Options"="K76", "Flags"=0, "Help"="Selects the order in which the signal is displayed in the honeycomb.\n\nAvailable Repeated Capabilities:\nSerialBus: SB1, SB2, SB3, SB4\r\n\nRemote-control command(s):\nBUS<m>:CXPI:DORD"}, {"Level"=3, "Class Only"=FALSE, "Identifier"="RSSCOPE_ATTR_PROTOCOL_CXPI_AVERAGE_BIT_RATE_ENABLED", "Descriptive Name"="Protocol CXPI Average Bit Rate Enabled", "Data Type"=3, "Command"="BUS{SerialBus}:CXPI:BITR:ENAB", "Access"=2, "Range Table"="", "Read Callback"="", "Write Callback"="", "Supported Models"="", "Instrument Options"="K76", "Flags"=0, "Help"="Enables the manual setting of a bit rate.\n\nAvailable Repeated Capabilities:\nSerialBus: SB1, SB2, SB3, SB4\r\n\nRemote-control command(s):\nBUS<m>:CXPI:BITRate:ENABle"}, {"Level"=3, "Class Only"=FALSE, "Identifier"="RSSCOPE_ATTR_PROTOCOL_CXPI_BIT_RATE_VALUE", "Descriptive Name"="Protocol CXPI Bit Rate Value", "Data Type"=0, "Command"="BUS{SerialBus}:CXPI:BITR:VAL", "Access"=2, "Range Table"="RsScope_rngCXPIBitRateValue", "Read Callback"="", "Write Callback"="", "Supported Models"="", "Instrument Options"="K76", "Flags"=0, "Help"="Sets the number of transmitted bits per second.\n\nAvailable Repeated Capabilities:\nSerialBus: SB1, SB2, SB3, SB4\r\n\nRemote-control command(s):\nBUS<m>:CXPI:BITRate:VALue"}, {"Level"=3, "Class Only"=FALSE, "Identifier"="RSSCOPE_ATTR_PROTOCOL_CXPI_MEASURED_BIT_RATE", "Descriptive Name"="Protocol CXPI Measured Bit Rate", "Data Type"=0, "Command"="BUS{SerialBus}:CXPI:RES:BITR?", "Access"=0, "Range Table"="", "Read Callback"="", "Write Callback"="", "Supported Models"="", "Instrument Options"="K76", "Flags"=0, "Help"="Queries the measured average bit rate, which is calculated.\n\nAvailable Repeated Capabilities:\nSerialBus: SB1, SB2, SB3, SB4\r\n\nRemote-control command(s):\nBUS<m>:CXPI:RESult:BITRate?"}, {"Level"=3, "Class Only"=FALSE, "Identifier"="RSSCOPE_ATTR_PROTOCOL_CXPI_EXPECTED_IBS_MIN", "Descriptive Name"="Protocol CXPI Expected IBS Min", "Data Type"=0, "Command"="BUS{SerialBus}:CXPI:IBS:MIN", "Access"=2, "Range Table"="RsScope_rngCXPIExpectedIBS", "Read Callback"="", "Write Callback"="", "Supported Models"="", "Instrument Options"="K76", "Flags"=0, "Help"="Sets the minimum for the inter-byte-space range.\n\nAvailable Repeated Capabilities:\nSerialBus: SB1, SB2, SB3, SB4\r\n\nRemote-control command(s):\nBUS<m>:CXPI:IBS:MIN"}, {"Level"=3, "Class Only"=FALSE, "Identifier"="RSSCOPE_ATTR_PROTOCOL_CXPI_EXPECTED_IBS_MAX", "Descriptive Name"="Protocol CXPI Expected IBS Max", "Data Type"=0, "Command"="BUS{SerialBus}:CXPI:IBS:MAX", "Access"=2, "Range Table"="RsScope_rngCXPIExpectedIBS", "Read Callback"="", "Write Callback"="", "Supported Models"="", "Instrument Options"="K76", "Flags"=0, "Help"="Sets the maximum for the inter-byte-space range.\n\nAvailable Repeated Capabilities:\nSerialBus: SB1, SB2, SB3, SB4\r\n\nRemote-control command(s):\nBUS<m>:CXPI:IBS:MAX"}, {"Level"=3, "Class Only"=FALSE, "Identifier"="RSSCOPE_ATTR_PROTOCOL_CXPI_EXPECTED_IFS_MIN", "Descriptive Name"="Protocol CXPI Expected IFS Min", "Data Type"=0, "Command"="BUS{SerialBus}:CXPI:IFS:MIN", "Access"=2, "Range Table"="RsScope_rngCXPIExpectedIFSMin", "Read Callback"="", "Write Callback"="", "Supported Models"="", "Instrument Options"="K76", "Flags"=0, "Help"="Sets the minimum for the inter-frame-space range.\n\nAvailable Repeated Capabilities:\nSerialBus: SB1, SB2, SB3, SB4\r\n\nRemote-control command(s):\nBUS<m>:CXPI:IFS:MIN"}, {"Level"=3, "Class Only"=FALSE, "Identifier"="RSSCOPE_ATTR_PROTOCOL_CXPI_EXPECTED_IFS_MAX", "Descriptive Name"="Protocol CXPI Expected IFS Max"
